vi "Read Waveform.vi"(7 "Waveform Start (1)":i32=1, 8 "error in (no error)":errorcluster {"code" format="%.0x"}, 9 "Waveform End (10000)":i32=10000, 10 "Source (Channel 1)":string(combo)="CH1", 11 "VISA Resource Name":refnum<visa-resource-name>) -> (0 "error out":errorcluster {"code" format="%.0x"}, 1 "X Increment":dbl format="%.2e", 2 "Initial X":dbl format="%.2e", 3 "VISA Resource Name Out":refnum<visa-resource-name>, 4 "Waveform Array":dbl[](array[numeric]) format="%.2f", 5 "Actual Points":u32)   [LabVIEW 2010, in "Tektronix TDS 3000 Series.lvlib"]
doc: "This VI initiates a new acquisition, retrieves the waveform (starting and ending at Waveform Start and Waveform End,respectively), scales the data, and returns an array of DBLs.\n\nNote:\n(1) In order for this VI to work the waveform must be displayed on the instrument.\n(2) This is only used with Normal and Average Acquisition Types\n(3) The instrument will return an error if you attempt to read more points than stored on the instrument. Set the desired record length in the Configure Acquisition Record VI."
uses:
  <instrlib>/Tektronix TDS 3000 Series/Tektronix TDS 3000 Series.lvlib
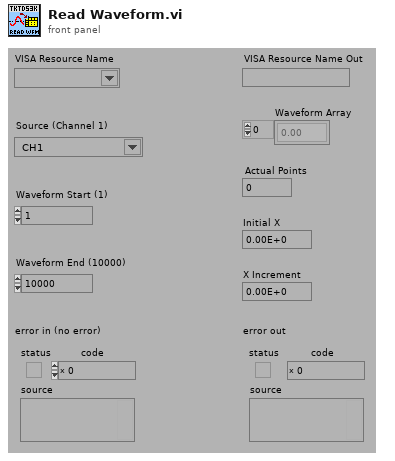
[diagram p1: front panel]
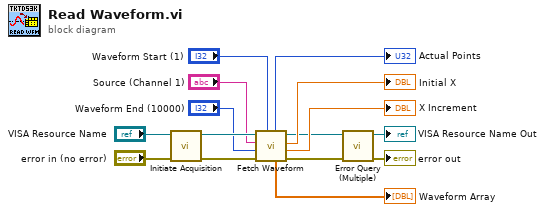
[diagram p0: block diagram]
diagram:
  n1 = call <instrlib>:"Initiate Acquisition.vi"("error in (no error)"="error in (no error)", "VISA Resource Name"="VISA Resource Name") -> ("error out"=w12:errorcluster, "VISA Resource Name Out"=w13:refnum<visa-resource-name>)  [unwired: 8 in]
  n2 = call <instrlib>:"Fetch Waveform.vi"("Waveform Start (1)"="Waveform Start (1)", "error in (no error)"=w12, "Waveform End (10000)"="Waveform End (10000)", "Source (Channel 1)"="Source (Channel 1)", "VISA Resource Name"=w13) -> ("error out"=w4:errorcluster, "X Increment"=→"X Increment":dbl, "Initial X"=→"Initial X":dbl, "VISA Resource Name Out"=w3:refnum<visa-resource-name>, "Waveform Array"=→"Waveform Array":dbl[], "Actual Points"=→"Actual Points":u32)  [unwired: 1 in]
  n3 = call <instrlib>:"Error Query (Multiple).vi"("error in (no error)"=w4, "VISA Resource Name"=w3) -> ("error out"=→"error out":errorcluster, "VISA Resource Name Out"=→"VISA Resource Name Out":refnum<visa-resource-name>)  [unwired: 6 in, 2 out]
